vi "Set camera parameter.vi"(8 "error in (no error)":errorcluster, 11 "DAQCascade512II in":refnum<class "DAQCascade512II.lvclass">) -> (0 "error out":errorcluster, 3 "DAQCascade512II out":refnum<class "DAQCascade512II.lvclass">)   [LabVIEW 2012, in "DAQCascade512II.lvclass"]
uses:
  DAQCascade512II.lvclass
  DAQCascade512II.lvclass/DAQCascade512II.ctl
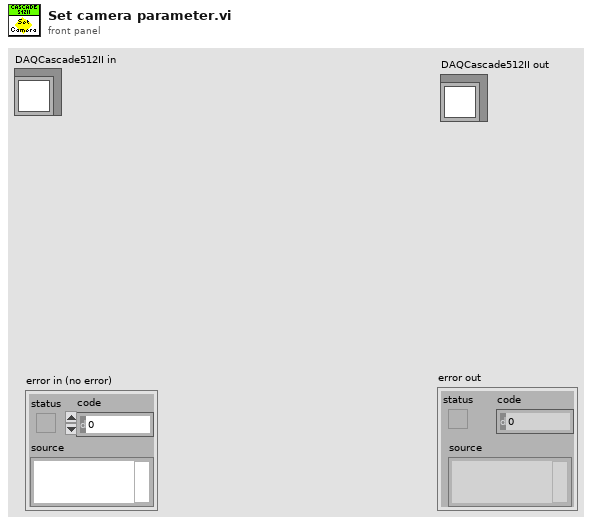
[diagram p1: front panel]
types:
  T1 = typedef "DAQCascade512II.lvclass/Exposure (sec).ctl" = dbl
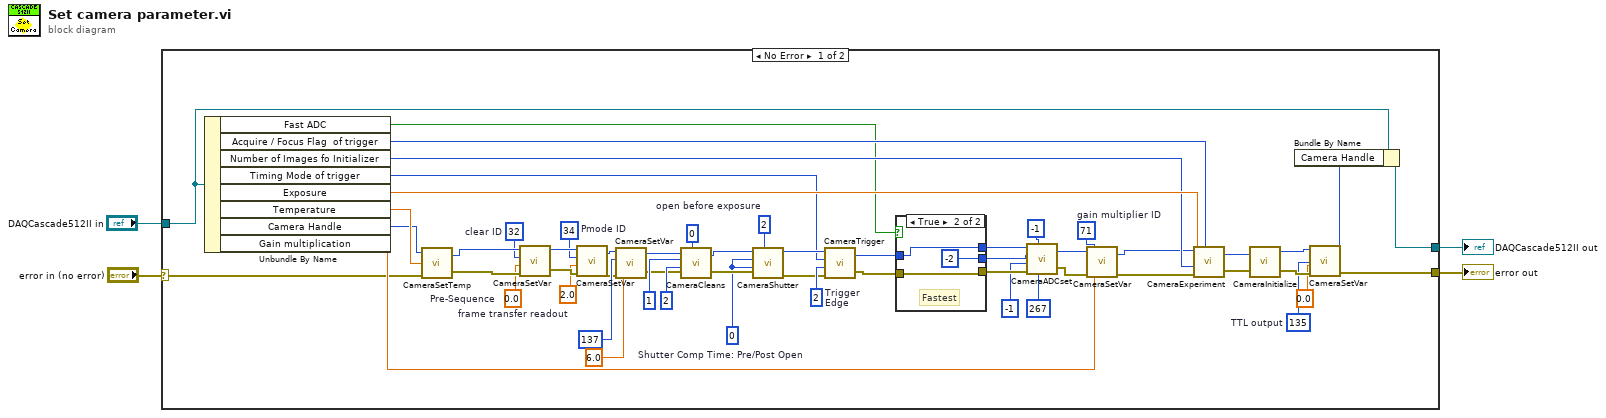
[diagram p0: block diagram]
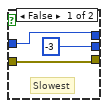
[diagram p2: hidden frame]
diagram:
  n1 = case shown="No Error" "error in (no error)" {
    selector: "error in (no error)" -> [w6 w68]
    tunnel: [w5 w68] -> w4
    tunnel: [w22 w67] -> w3
    tunnel: "DAQCascade512II in" -> [w21 w67]
    frame No Error {
      w16 = u32 135  # TTL output
      w32 = 2.0  # frame transfer readout
      w33 = u32 34  # Pmode ID
      w34 = 0.0  # Pre-Sequence
      w35 = u32 32  # clear ID
      w41 = u32 71  # gain multiplier ID
      w53 = u32 0  # Shutter Comp Time: Pre/Post Open
      w51 = u32 2  # Trigger  Edge
      w20 = u32 2  # open before exposure
      n2 = Unbundle By Name(w21) -> ("Fast ADC"=w31:bool, "Acquire / Focus Flag  of trigger"=w55:u32, "Number of Images fo Initializer"=w52:u32, "Timing Mode of trigger"=w48:u32, "Exposure"=w54:T1, "Temperature"=w56:dbl, "Camera Handle"=w44:u32, "Gain multiplication"=w40:dbl)
      n3 = call <userlib>:"CameraSetTemp.vi"("error in (no error)"=w6, "Temperature"=w56, "Camera Handle"=w44) -> ("error out"=w36:errorcluster, "Camera Handle"=w37:u32)
      n4 = call <userlib>:"CameraSetVar.vi"("error in"=w36, "Value"=w34, "Parameter ID"=w35, "Camera Handle"=w37) -> ("error out"=w39:errorcluster, "CameraHandle"=w38:u32)
      n5 = call <userlib>:"CameraSetVar.vi"("error in"=w39, "Value"=w32, "Parameter ID"=w33, "Camera Handle"=w38) -> ("error out"=w10:errorcluster, "CameraHandle"=w13:u32)
      n6 = call <userlib>:"CameraSetVar.vi"("error in"=w10, "Value"=6.0, "Parameter ID"=u32 137, "Camera Handle"=w13) -> ("error out"=w9:errorcluster, "CameraHandle"=w8:u32)
      n7 = call <userlib>:"CameraCleans.vi"("Camera Handle"=w8, "Number of Clears"=u32 1, "Number of Strips Per Clear"=u32 2, "error in"=w9, "Continuous Clears"=u32 0) -> ("Camera Handle"=w59:u32, "error out"=w60:errorcluster)
      n8 = call <userlib>:"CameraShutter.vi"("Camera Handle"=w59, "Shutter Comp Time: Pre Open"=w53, "Shutter Comp Time: Post Open"=w53, "error in"=w60, "Shutter State"=w20) -> ("Camera Handle"=w50:u32, "error out"=w49:errorcluster)
      n9 = call <userlib>:"CameraTrigger.vi"("error in"=w49, "Trigger Edge"=w51, "Timing Mode"=w48, "Camera Handle"=w50) -> ("error out"=w30:errorcluster, "Camera Handle"=w28:u32)
      n10 = case shown="True" w31 {
        tunnel: [-3 -2] -> w19
        tunnel: [w62 w64] -> w29
        tunnel: w30 -> [w62 w64]
        tunnel: w28 -> [w61 w65]
        tunnel: [w61 w65] -> w27
        frame False {
          # "Slowest"
        }
        frame True {
          # "Fastest"
        }
      }
      n11 = call <userlib>:"CameraADCset.vi"("ADC offset"=267, "Read Out port"=-1, "error in (no error)"=w29, "ADC Gain"=-1, "ADC Speed"=w19, "Camera Handle"=w27) -> ("error out"=w23:errorcluster, "Camera Handle"=w7:u32)
      n12 = call <userlib>:"CameraSetVar.vi"("error in"=w23, "Value"=w40, "Parameter ID"=w41, "Camera Handle"=w7) -> ("error out"=w43:errorcluster, "CameraHandle"=w42:u32)
      n13 = call <userlib>:"CameraExperiment.vi"("Acquire / Focus Flag"=w55, "error in"=w43, "Number of Images"=w52, "Exposure (sec)"=w54, "Camera Handle"=w42) -> ("error out"=w57:errorcluster, "Camera Handle"=w58:u32)  [unwired: 1 in]
      n14 = call <userlib>:"CameraInitialize.vi"("error in"=w57, "Camera Handle"=w58) -> ("error out"=w17:errorcluster, "Camera Handle"=w18:u32)
      n15 = call <userlib>:"CameraSetVar.vi"("error in"=w17, "Value"=0.0, "Parameter ID"=w16, "Camera Handle"=w18) -> ("error out"=w5:errorcluster, "CameraHandle"=w14:u32)
      n16 = Bundle By Name(cluster=w21, "Camera Handle"=w14) -> (w22:refnum<class "DAQCascade512II.lvclass">)
    }
    frame Error {
    }
  }
  "error out" <- w4
  "DAQCascade512II out" <- w3
